vi "get hot goal.vi"() -> (0 "Goals Used":i32, 1 "Hot Goal Found":bool, 3 "Right Hot":bool)   [LabVIEW 2013]
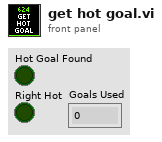
[diagram p1: front panel]
types:
  T1 = typedef "Goal Info.ctl" = cluster{"Found?":bool, "Target Center":cluster{"X":dbl, "Y":dbl}, "Distance (ft)":dbl, "Hot?":bool, "Left?":bool, "Camera":i16}
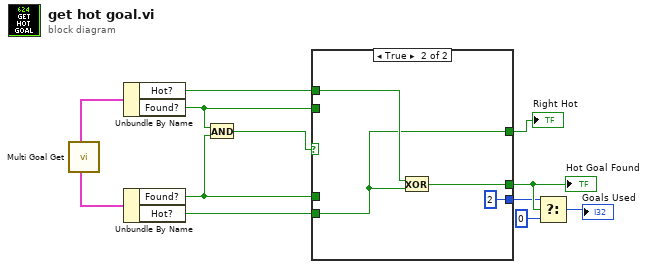
[diagram p0: block diagram]
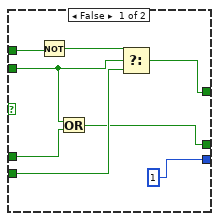
[diagram p2: hidden frame]
diagram:
  n1 = call "Multi Goal Get.vi"() -> ("R Target"=w11:T1, "L Target"=w12:T1)  [unwired: 4 in, 6 out]
  n2 = Unbundle By Name(w12) -> ("Hot?"=w10:bool, "Found?"=w6:bool)
  n3 = Unbundle By Name(w11) -> ("Found?"=w5:bool, "Hot?"=w9:bool)
  n4 = And(x=w6, y=w5) -> (x .and. y?=w8:bool)
  n5 = case shown="True" w8 {
    tunnel: w10 -> [w20 w24]
    tunnel: w9 -> [w17 w22]
    tunnel: [w14 w23] -> w4
    tunnel: [w18 w22] -> w7
    tunnel: w6 -> [w16 _]
    tunnel: w5 -> [w15 _]
    tunnel: [1 2] -> w3
    frame False {
      n6 = Not(x=w20) -> (.not. x?=w19:bool)
      n7 = Or(x=w16, y=w15) -> (x .or. y?=w14:bool)
      n8 = Select(t=w19, s=w16, f=w17) -> (s? t:f=w18:bool)
    }
    frame True {
      n9 = Exclusive Or(1:w22, 2:w24) -> (0:w23:bool)
    }
  }
  "Hot Goal Found" <- w4
  "Right Hot" <- w7
  n10 = Select(t=w3, s=w4, f=0) -> (s? t:f=→"Goals Used":i32)
